vi "lia_fpga3.vi"() -> ()   [LabVIEW 2009]
uses:
  <vilib>/Platform/TimedLoop/XDataNode/XDataNode.xnode
  <vilib>/Platform/TimedLoop/XDataNode/loadlvalarms.vi
  <vilib>/Platform/TimedLoop/XDataNode/timing_clust.ctl
  <vilib>/Platform/TimedLoop/XDataNode/nitl_modes.ctl
  <vilib>/Platform/TimedLoop/XDataNode/wakeup.ctl
  <vilib>/rvi/DataTransferAndStorage/Container/XNode/niFpgaContainer.xnode
  <vilib>/rvi/FIFO/Fifo_Resource/nirvififoUniquifyingName.vi
  <vilib>/eio/EIONode/EIONode.xnode
  <vilib>/rvi/eio/nirviEIOImplementation/nirviEIOImplementation.xnode
  <vilib>/rvi/eio/common/nirviEmuTemplateMethod_noerrors.vi
  <vilib>/rvi/eio/common/nirviEmuClasses.ctl
  <vilib>/rvi/LocalResourceManager/LocalResourceManager.xnode
  <vilib>/rvi/eio/common/nirviEmuReportErrorAndStop.vi
  <vilib>/rvi/DataTransferAndStorage/Container/Common/niFpgaContainerSetEmuInfo.vi
  <vilib>/rvi/DataTransferAndStorage/Container/Common/niFpgaContainerState.ctl
  <vilib>/rvi/DataTransferAndStorage/Container/Common/niFpgaDataTypeControl.ctl
  <vilib>/rvi/DataTransferAndStorage/Container/Common/niFpgaContainerImplementationControl.ctl
  <vilib>/rvi/DataTransferAndStorage/Container/Common/niFpgaContainerArbitrationOptionsControl.ctl
  <vilib>/rvi/DataTransferAndStorage/Container/Common/niFpgaTransferTypeControl.ctl
  <vilib>/rvi/DataTransferAndStorage/Container/Common/niFpgaContainerInitializationParameters.ctl
  <vilib>/rvi/DataTransferAndStorage/Container/Common/niFpgaContainerMetaDataKey.ctl
  <vilib>/Platform/TimedLoop/XDataNode/XDNodeRunTimeDep.lvlib
panel:
  out "X_fpga":i16
  out "Y_fpga":i16
  out "Y_filt":i32
  out "X_filt":i32
  in  "stop 3":bool
  in  "Phase Shift Cos":u32
  in  "beta":i32
  in  "stop 2":bool
  in  "stop":bool
  out "Actual Gen Rate (ticks)":u32
  in  "Update Rate (ticks)":u32
  out "Accumulator Value":u32
  in  "Signal Amplitude":u16
  in  "Phase Shift":u32
  in  "Accumulator Increment":u32
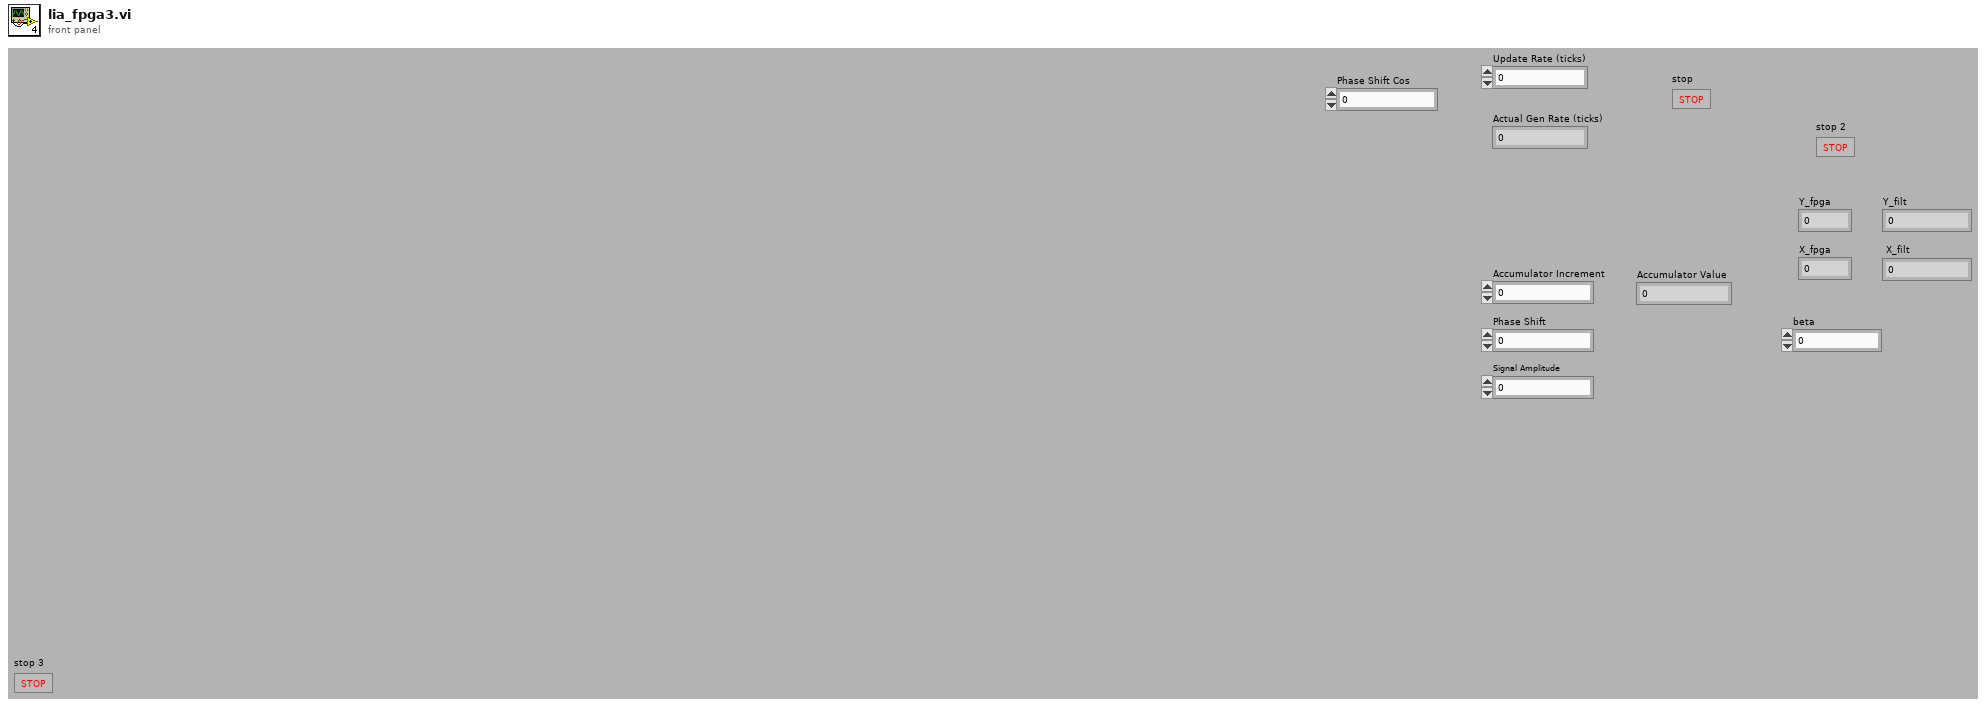
[diagram p1: front panel]
types:
  T1 = typedef "XDNodeRunTimeDep.lvlib/timing_clust.ctl" = cluster{"Expected End [f-1]":u64, "Actual End [f-1]":u64, "Finished Late? [f-1]":bool, "Expected End [i-1]":u64, "Actual End [i-1]":u64, "Finished Late? [i-1]":bool, "Expected Start [i]":u64, "Actual Start [i]":u64, "Expected Start [f]":u64, "Actual Start [f]":u64, "Source Name":string, "Structure Name":string, "Period":i64, "Deadline":i64, "Offset":i64, "Start":i64, "Priority":i32, "Timeout":i32, "Mode":T2, "Wakeup Reason":T3, "Error":errorcluster, "Source Type":string, "Secondary Source Type":string, "Global End Time":u64, "Global Start Time":u64, "Frame Duration":u64, "Iteration Duration":u64, "Assigned CPU":i32, "I/O Scan Engine Mode":u32}
  T2 = typedef "XDNodeRunTimeDep.lvlib/nitl_modes.ctl" = enum32{"No Change", "Process missed periods, maintain original phase", "Discard missed periods, maintain original phase", "Process missed periods, ignore original phase", "Discard missed periods, ignore original phase"}
  T3 = typedef "XDNodeRunTimeDep.lvlib/wakeup.ctl" = enum32{"Normal", "Aborted", "Asynchronous wakeup", "Timing source error", "Timed loop error", "Timeout"}
  T4 = typedef "nirviEmuClasses.ctl" = enum16{"IO Read", "IO Write", "Method", "Property Read", "Property Write"}
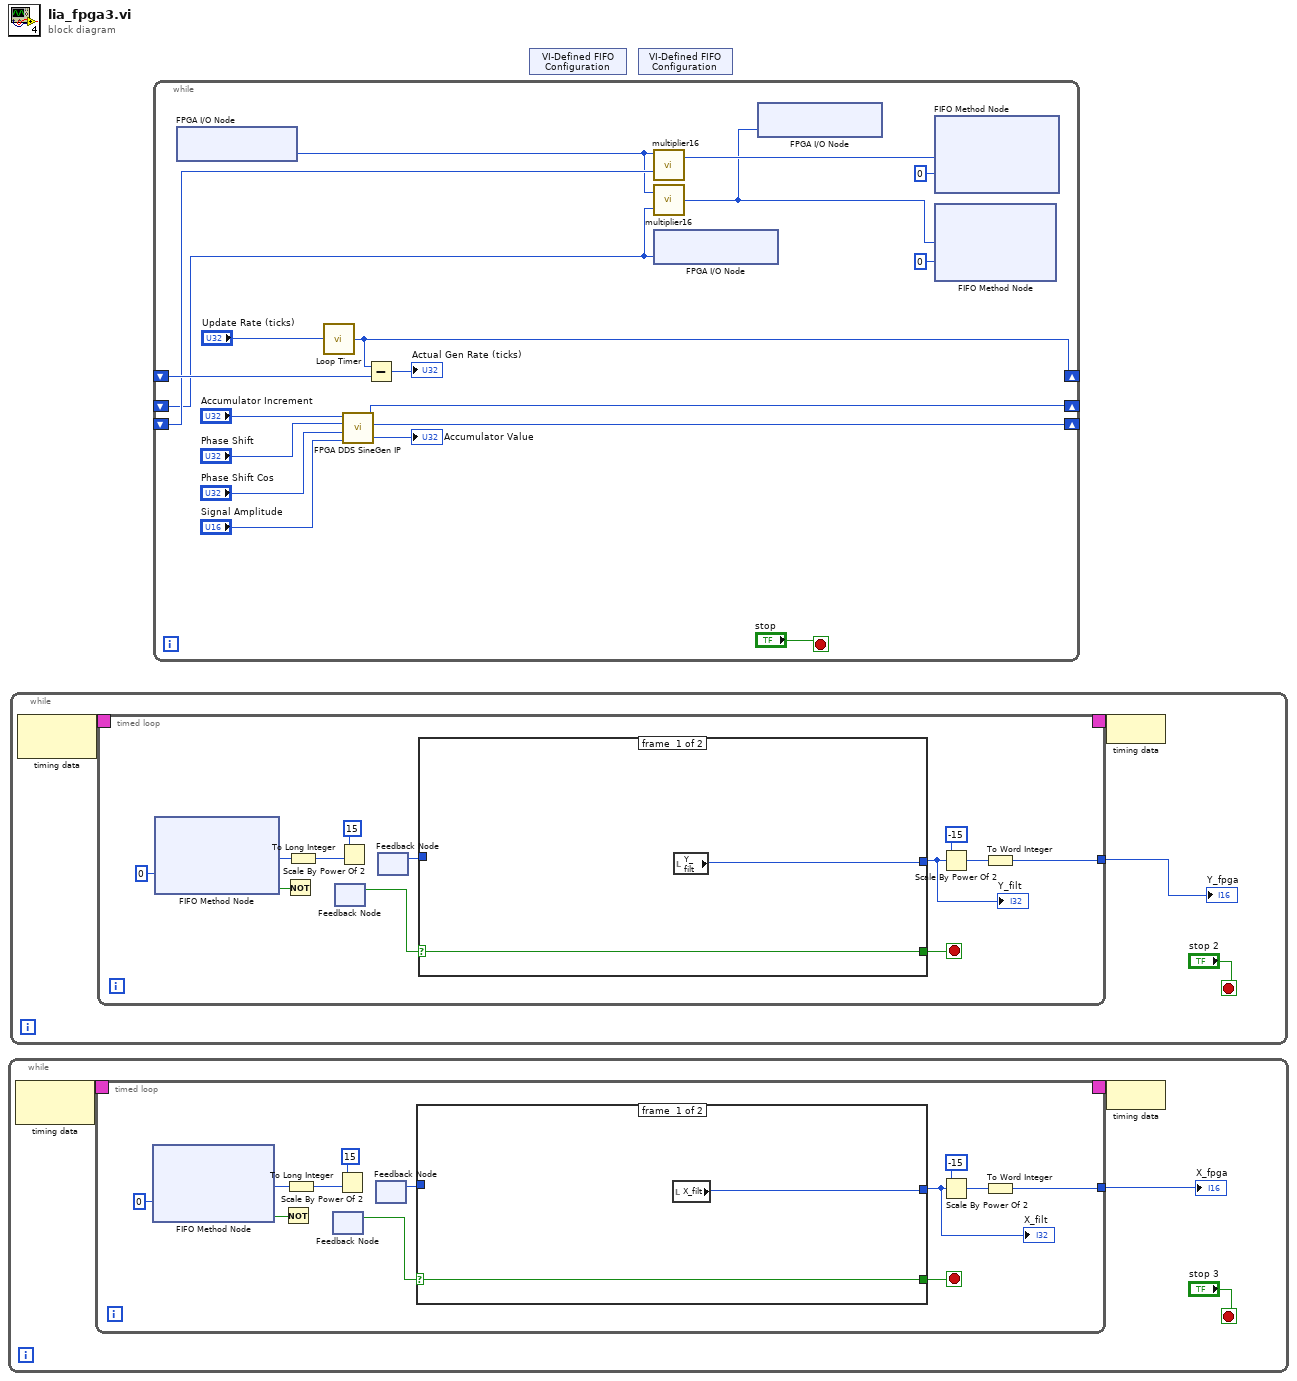
[diagram p0: block diagram]
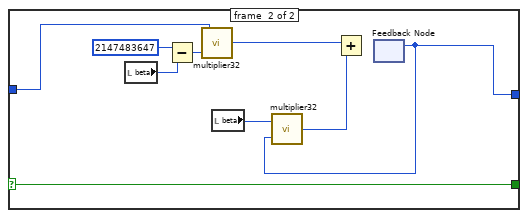
[diagram p2: hidden frame]
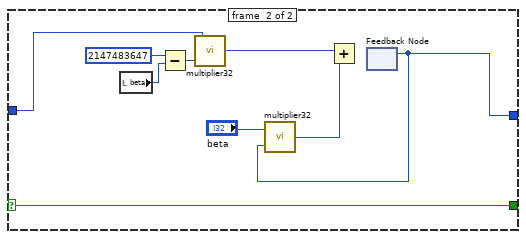
[diagram p3: hidden frame]
diagram:
  n1 = while {
    stop <- "stop 3" stop-if-true
    n2 = node-c288() -> (w4:T1)  [unwired: 1 in]
    n3 = timed-loop {
      timing: w4 -> [_]
      timing-out: [_] -> w3
      tunnel: [w11] -> w1
      stop <- w14 stop-if-true
      n4 = xnode ("FIFO Method Node")("Timeout"=0) -> ("Element"=w12:i16, "Timed Out?"=w17:bool)  [unwired: 1 in, 1 out]
      n5 = Not(x=w17) -> (.not. x?=w16:bool)
      n6 = To Long Integer(number=w12) -> (32bit integer=w10:i32)
      n7 = feedback #1() -> (w15:bool)  [unwired: 1 in]
      n8 = Scale By Power Of 2(n=i16 15, x=w10) -> (x*2^n=w9:i32)
      n9 = feedback #2() -> (w13:i32)  [unwired: 1 in]
      n10 = case shown="True" w15 {
        selector: w15 -> [w19 w30]
        tunnel: [w20 w23] -> w5
        tunnel: [w19 w30] -> w14
        tunnel: w13 -> [_ w24]
        frame #0 {
          n11 = local read "X_filt"() -> (w20:i32)
        }
        frame #1 {
          n12 = local read "beta"() -> (w22:i32)
          n13 = Subtract(x=2147483647, y=w22) -> (x-y=w26:i32)
          n14 = call "multiplier32.vi"("Y"=w26, "X"=w24) -> ("XY"=w27:i32)
          n15 = local read "beta"() -> (w21:i32)
          n16 = feedback #3() -> (w23:i32)  [unwired: 1 in]
          n17 = call "multiplier32.vi"("Y"=w23, "X"=w21) -> ("XY"=w25:i32)
          n18 = Add(x=w27, y=w25) -> (x+y=w28:i32)
        }
      }
      "X_filt" <- w5
      n19 = Scale By Power Of 2(n=i16 -15, x=w5) -> (x*2^n=w6:i32)
      n20 = To Word Integer(number=w6) -> (16bit integer=w11:i16)
    }
    "X_fpga" <- w1
    n21 = node-c288(w3) -> ()
  }
  n22 = while {
    stop <- "stop 2" stop-if-true
    n23 = node-c288() -> (w86:T1)  [unwired: 1 in]
    n24 = timed-loop {
      timing: w86 -> [_]
      timing-out: [_] -> w85
      tunnel: [w93] -> w83
      stop <- w96 stop-if-true
      n25 = xnode ("FIFO Method Node")("Timeout"=0) -> ("Element"=w94:i16, "Timed Out?"=w99:bool)  [unwired: 1 in, 1 out]
      n26 = Not(x=w99) -> (.not. x?=w98:bool)
      n27 = To Long Integer(number=w94) -> (32bit integer=w92:i32)
      n28 = feedback #4() -> (w97:bool)  [unwired: 1 in]
      n29 = Scale By Power Of 2(n=i16 15, x=w92) -> (x*2^n=w91:i32)
      n30 = feedback #5() -> (w95:i32)  [unwired: 1 in]
      n31 = case shown="True" w97 {
        selector: w97 -> [w101 w112]
        tunnel: [w102 w103] -> w87
        tunnel: [w101 w112] -> w96
        tunnel: w95 -> [_ w104]
        frame #0 {
          n32 = local read "Y_filt"() -> (w102:i32)
        }
        frame #1 {
          n33 = local read "beta"() -> (w110:i32)
          n34 = Subtract(x=2147483647, y=w110) -> (x-y=w107:i32)
          n35 = call "multiplier32.vi"("Y"=w107, "X"=w104) -> ("XY"=w108:i32)
          n36 = feedback #6() -> (w103:i32)  [unwired: 1 in]
          n37 = call "multiplier32.vi"("Y"=w103, "X"="beta") -> ("XY"=w106:i32)
          n38 = Add(x=w108, y=w106) -> (x+y=w109:i32)
        }
      }
      "Y_filt" <- w87
      n39 = Scale By Power Of 2(n=i16 -15, x=w87) -> (x*2^n=w88:i32)
      n40 = To Word Integer(number=w88) -> (16bit integer=w93:i16)
    }
    "Y_fpga" <- w83
    n41 = node-c288(w85) -> ()
  }
  n42 = while {
    shift-right: [w180] -> _
    shift-left: _ -> [w168]
    shift-right: [w179] -> _
    shift-left: _ -> [w177]
    shift-right: [w173] -> _
    shift-left: _ -> [w169]
    stop <- "stop" stop-if-true
    n43 = xnode "FPGA I/O Node"() -> ("Connector0/AI0"=w167:i16)  [unwired: 1 in, 1 out]
    n44 = call "Loop Timer"("Count(Ticks)"="Update Rate (ticks)") -> ("Tick Count(Ticks)"=w179:u32)
    n45 = call "FPGA DDS SineGen IP.vi"("Signal Amplitude (x 2^15)"="Signal Amplitude", "Phase Shift Cos"="Phase Shift Cos", "Phase Shift"="Phase Shift", "Accumulator Increment"="Accumulator Increment") -> ("Accumulator Value"=→"Accumulator Value":u32, "Cos output"=w173:i16, "Sin output"=w180:i16)  [unwired: 5 in]
    n46 = Subtract(x=w179, y=w177) -> (x-y=→"Actual Gen Rate (ticks)":u32)
    n47 = call "multiplier16.vi"("Y"=w169, "X"=w167) -> ("XY"=w166:i16)
    n48 = call "multiplier16.vi"("Y"=w168, "X"=w167) -> ("XY"=w165:i16)
    n49 = xnode "FPGA I/O Node"("Connector0/AO0"=w168) -> ()  [unwired: 1 in, 1 out]
    n50 = xnode "FPGA I/O Node"("Connector0/AO1"=w165) -> ()  [unwired: 1 in, 1 out]
    n51 = xnode ("FIFO Method Node")("Element"=w166, "Timeout"=0) -> ()  [unwired: 1 in, 2 out]
    n52 = xnode ("FIFO Method Node")("Element"=w165, "Timeout"=0) -> ()  [unwired: 1 in, 2 out]
  }
  n53 = xnode "VI-Defined FIFO Configuration"() -> ()  [unwired: 1 out]
  n54 = xnode "VI-Defined FIFO Configuration"() -> ()  [unwired: 1 out]
